vi "ASK_return10.vi"(8 "error in (no error)":errorcluster caption="错误输入（无错误）", 10 "inputdata":i32[](array[numeric]), 11 "PathIn":path) -> (0 "error out":errorcluster caption="错误输出", 2 "outputdata":i32[](array[numeric]), 3 "PathOut":path)   [LabVIEW 2015]
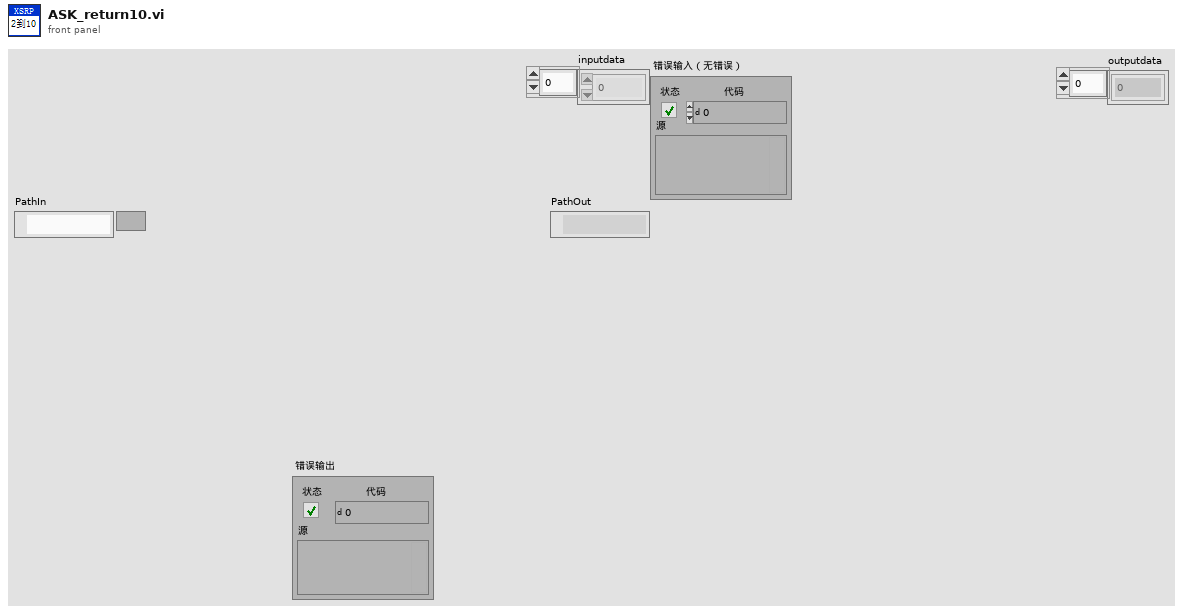
[diagram p1: front panel]
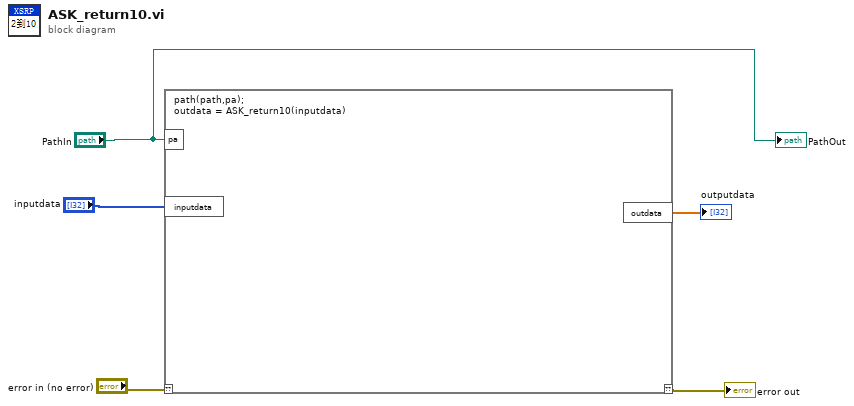
[diagram p0: block diagram]
diagram:
  n1 = script code="path(path,pa);\noutdata = ASK_return10(inputdata)"("??"="error in (no error)", "pa"="PathIn", "inputdata"="inputdata") -> ("??"=→"error out":errorcluster, "outdata"=→"outputdata":cdb[])
  "PathOut" <- "PathIn"
